vi "Read Mode.vi"(8 "Error In":errorcluster, 11 "Session In":refnum<class "Session.lvclass">) -> (0 "Error Out":errorcluster, 2 "Mode":T1, 3 "Sesssion Out":refnum<class "Session.lvclass">)   [LabVIEW 2017, in "LabSSH2.lvlib" / "Session.lvclass"]
uses:
  Session.lvclass
  Typedefs/Modes.ctl
  Session.lvclass/Session.ctl
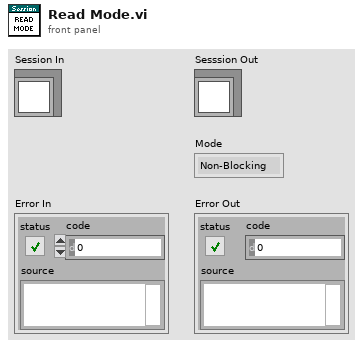
[diagram p1: front panel]
types:
  T1 = typedef "LabSSH2.lvlib/Session.lvclass/Modes.ctl" = enum32{"Non-Blocking", "Blocking"}
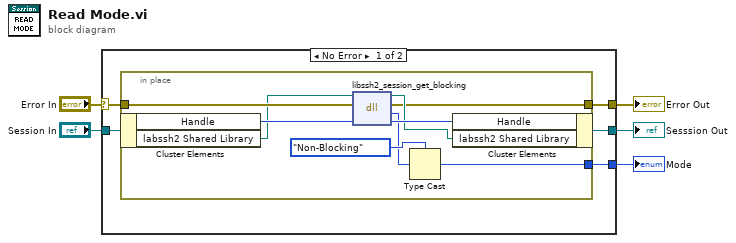
[diagram p0: block diagram]
diagram:
  n1 = case shown="No Error" "Error In" {
    selector: "Error In" -> [w9 w21]
    tunnel: [w10 w21] -> w4
    tunnel: "Session In" -> [w8 w20]
    tunnel: [w7 w20] -> w2
    tunnel: [w6 _] -> w1
    frame No Error {
      n2 = in-place {
        in-place-border: [w14] -> w10
        in-place-border: w9 -> [w19]
        in-place-border: [w11] -> w6
        n3 = in-place-cluster #1(w8) -> ("Handle"=w18:u64, "labssh2 Shared Library"=w16:path)
        n4 = dll-call lib="D:/Users/cfield/Code/Field R&D Services/SSH/LabSSH2/LabVIEW/trunk/src/LabSSH2/Private/labssh2.*" fn="libssh2_session_get_blocking"(path in=w16, error in=w19, "session"=w18) -> (path out=w15:path, error out=w14:errorcluster, "result"=w12:i32, "session"=w17:u64)  [unwired: 1 in]
        n5 = Type Cast(type=Modes."Non-Blocking" ("Mode"), x=w12) -> (*(type *) &x=w11:T1)
        n6 = in-place-cluster #1("Handle"=w17, "labssh2 Shared Library"=w15) -> (w7:refnum<class "Session.lvclass">)
      }
    }
    frame Error {
    }
  }
  "Sesssion Out" <- w2
  "Error Out" <- w4
  "Mode" <- w1
